vi "Init.vi"(8 "error in":errorcluster, 10 "Obj Entry":refnum<class "Object Entry.lvclass">, 11 "Transmit PDO in":refnum<class "TPDO Communication Parameter.lvclass">) -> (0 "error out":errorcluster, 3 "Transmit PDO out":refnum<class "TPDO Communication Parameter.lvclass">)   [LabVIEW 2020, in "CANopen.lvlib" / "TPDO Communication Parameter.lvclass"]
uses:
  TPDO Communication Parameter.lvclass
  Object Entry/Object Entry.lvclass
  Sub Object/Sub Object.lvclass/Sub Object.ctl
  TPDO Communication Parameter.lvclass/TPDO Communication Parameter.ctl
  Sub Object/Get Default Value.vi
  Sub Object/Default Value is null.vi
  Sub Object/Get Index.vi
  Sub Object/Get Sub Index.vi
  PDO Communication Parameter/PDO Communication Parameter.lvclass
  CANopen.lvlib
  Sub Object/Sub Object.lvclass
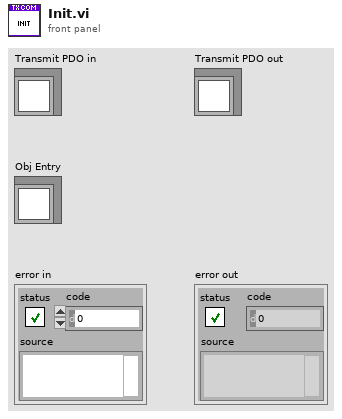
[diagram p1: front panel]
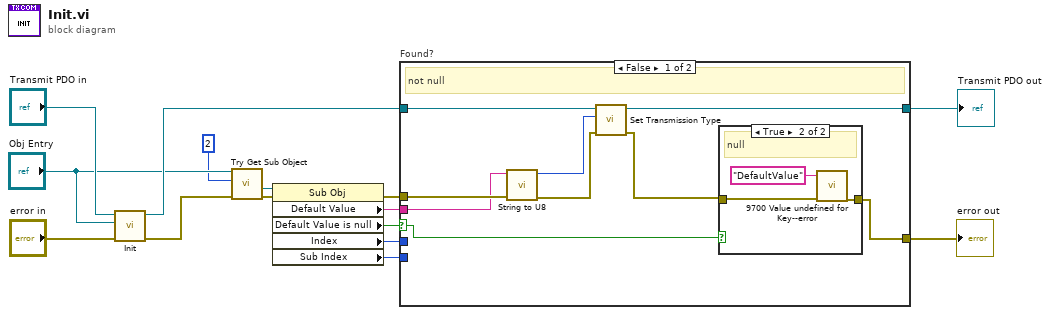
[diagram p0: block diagram]
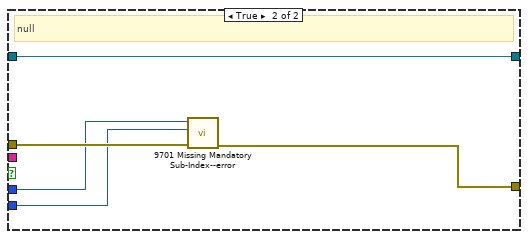
[diagram p3: hidden frame]
diagram:
  n1 = call-parent "Init.vi"("error in"="error in", "OD Entry"="Obj Entry", "PDO Communication Parameter in"="Transmit PDO in") -> ("error out"=w12:errorcluster, "PDO Communication Parameter out"=w10:refnum<class "TPDO Communication Parameter.lvclass">)  [unwired: 7 in]
  n2 = call "Try Get Sub Object.vi"("error in"=w12, "Sub Index"=u8 2, "Obj Entry in"="Obj Entry") -> ("error out"=w8:errorcluster, "Sub Object"=w6:refnum<class "Sub Object.lvclass">)  [unwired: 5 in, 2 out]
  n3 = property class="Sub Obj"(reference=w6, error in=w8) -> (error out=w7:errorcluster, "Default Value"=w4:string, "Default Value is null"=w5:bool, "Index"=w2:u16, "Sub Index"=w1:u8)  [unwired: 1 out]
  n4 = case "Found?" shown="False" w5 {
    selector: w5 -> [w19 _]
    tunnel: w10 -> [w24 w31]
    tunnel: [w23 w31] -> w13
    tunnel: [w21 w32] -> w14
    tunnel: w7 -> [w20 w33]
    tunnel: w4 -> [w18 _]
    tunnel: w2 -> [_ w30]
    tunnel: w1 -> [_ w29]
    frame False {
      # "not null"
      n5 = call "String to U8.vi"("error in"=w20, "Integer String"=w18) -> ("error out"=w16:errorcluster, "U8"=w17:u8)  [unwired: 8 in]
      n6 = call "Set Transmission Type.vi"("error in"=w16, "Transmission Type"=w17, "TPDO Communication Parameter in"=w24) -> ("error out"=w22:errorcluster, "TPDO Communication Parameter out"=w23:refnum<class "TPDO Communication Parameter.lvclass">)  [unwired: 7 in]
      n7 = case "null?" shown="True" w19 {
        tunnel: w22 -> [w25 w27]
        tunnel: [w25 w28] -> w21
        frame False {
          # "not null"
        }
        frame True {
          # "null"
          n8 = call "9700 Value undefined for Key--error.vi"("error in"=w27, "Argument"="DefaultValue" ("key")) -> ("error out"=w28:errorcluster)  [unwired: 9 in]
        }
      }
    }
    frame True {
      # "null"
      n9 = call "9701 Missing Mandatory Sub-Index--error.vi"("error in"=w33, "Sub-Index"=w29, "Index"=w30) -> ("error out"=w32:errorcluster)  [unwired: 8 in]
    }
  }
  "Transmit PDO out" <- w13
  "error out" <- w14
